vi "Read CAN Channels.vi"(7 "Peltier":T1, 8 "error in (no error)":errorcluster, 11 "Gas":T2) -> (0 "error out":errorcluster, 3 "CAN Values":dbl[](array[numeric]))   [LabVIEW 2014]
doc: "This VI is used as to not overload the CAN boards for acquiring data. The intent is to acquire one sample/second from the NI-DAQ hardware and one sample/5 seconds from the CAN boards. At the end of every 5 second cycle, fresh values are acquired. If in the middle of the 5 second wait, the last values are used. Please note that there is no timing inside this VI, it is solely dependent on the timing of the owning VI"
uses:
  CAN Communication/PAS/PAS.lvclass
  CAN Communication/PAS/Typedefs/Pressure Sensor.ctl
  CAN Communication/Peltier/Peltier.lvclass
  CAN Communication/Peltier/Typedefs/Peltier Temperature Sensors.ctl
  CAN Communication/PAS/Typedefs/Session Handle.ctl
  CAN Communication/Peltier/Typedefs/Session Handle.ctl
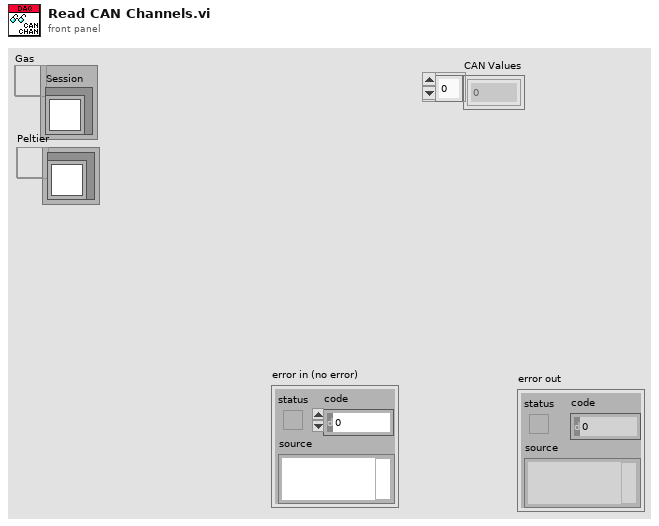
[diagram p1: front panel]
types:
  T1 = typedef "Peltier.lvclass/Session Handle.ctl" = refnum<data-value>
  T2 = typedef "PAS.lvclass/Session Handle.ctl" = refnum<data-value>
  T3 = typedef "Peltier.lvclass/Peltier Temperature Sensors.ctl" = u16
  T4 = typedef "PAS.lvclass/Pressure Sensor.ctl" = u16
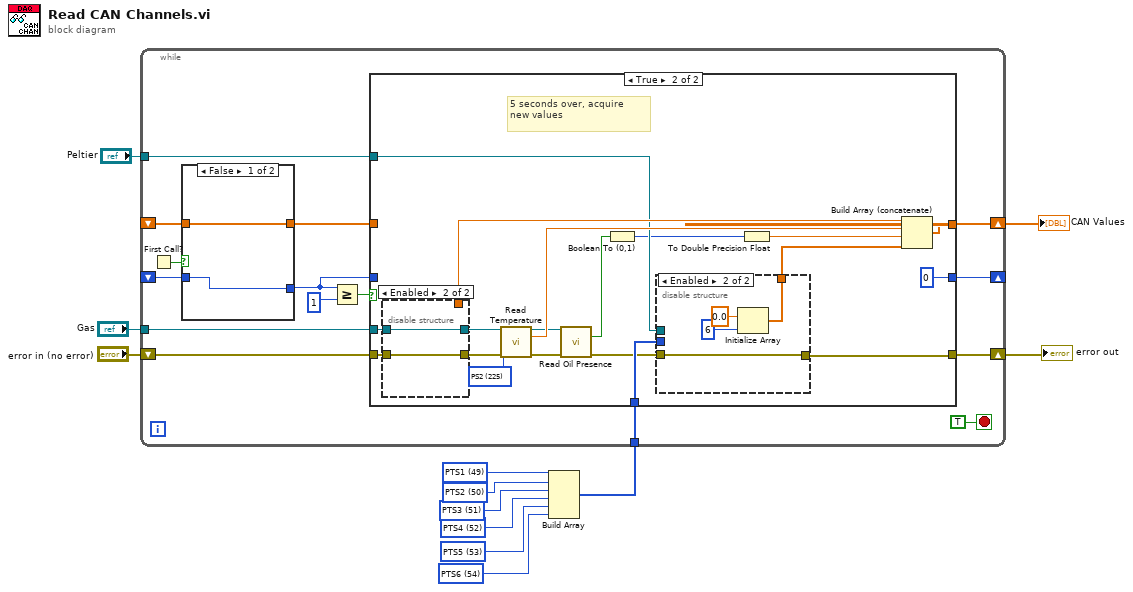
[diagram p0: block diagram]
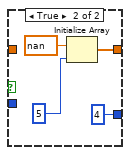
[diagram p2: hidden frame]
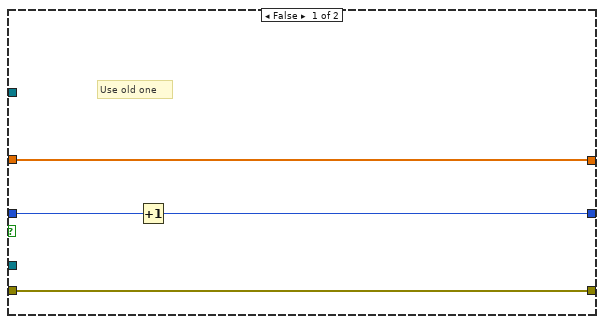
[diagram p3: hidden frame]
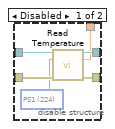
[diagram p4: hidden frame]
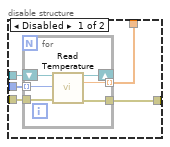
[diagram p5: hidden frame]
diagram:
  w2 = T3 54 items=["PTS1"=49, "PTS2"=50, "PTS3"=51, "PTS4"=52, "PTS5"=53, "PTS6"=54] ("Pelt Temp Sensors")
  w3 = T3 53 items=["PTS1"=49, "PTS2"=50, "PTS3"=51, "PTS4"=52, "PTS5"=53, "PTS6"=54] ("Pelt Temp Sensors")
  w4 = T3 52 items=["PTS1"=49, "PTS2"=50, "PTS3"=51, "PTS4"=52, "PTS5"=53, "PTS6"=54] ("Pelt Temp Sensors")
  w5 = T3 51 items=["PTS1"=49, "PTS2"=50, "PTS3"=51, "PTS4"=52, "PTS5"=53, "PTS6"=54] ("Pelt Temp Sensors")
  w6 = T3 50 items=["PTS1"=49, "PTS2"=50, "PTS3"=51, "PTS4"=52, "PTS5"=53, "PTS6"=54] ("Pelt Temp Sensors")
  w7 = T3 49 items=["PTS1"=49, "PTS2"=50, "PTS3"=51, "PTS4"=52, "PTS5"=53, "PTS6"=54] ("Pelt Temp Sensors")
  n1 = Build Array(w7, w6, w5, w4, w3, w2) -> (w1:T3[])
  n2 = while {
    tunnel: "Gas" -> [w23]
    shift-right: [w22] -> w10
    shift-left: _ -> [w19]
    shift-right: [w21] -> w9
    shift-left: "error in (no error)" -> [w24]
    shift-right: [w17] -> _
    shift-left: _ -> [w16]
    tunnel: "Peltier" -> [w14]
    tunnel: w1 -> [w13]
    stop <- TRUE stop-if-true
    n3 = First Call?() -> (First Call?: T/F=w20:bool)
    n4 = case shown="False" w20 {
      tunnel: [w29 w32] -> w15
      tunnel: [w28 4] -> w18
      tunnel: w19 -> [w29 _]
      tunnel: w16 -> [w28 _]
      frame False {
      }
      frame True {
        n5 = Initialize Array(nan ("element"), 5 ("dimension size")) -> (w32:dbl[])
      }
    }
    n6 = Greater Or Equal?(x=w18, y=1) -> (x >= y?=w26:bool)
    n7 = case shown="True" w26 {
      tunnel: w24 -> [w37 w56]
      tunnel: w23 -> [_ w55]
      tunnel: [w34 w49] -> w22
      tunnel: [w37 w45] -> w21
      tunnel: w18 -> [w36 _]
      tunnel: [w35 0] -> w17
      tunnel: w15 -> [w34 _]
      tunnel: w14 -> [_ w47]
      tunnel: w13 -> [_ w46]
      frame False {
        # "Use old one"
        n8 = Increment(x=w36) -> (x+1=w35:i32)
      }
      frame True {
        w52 = T4 225 items=["PS1"=224, "PS2"=225] ("Pressure Sensor")
        # "5 seconds over, acquire\nnew values"
        n9 = disable-structure shown="Enabled" {
          disable-tunnel: w56 -> [w62 w63]
          disable-tunnel: w55 -> [w60 w64]
          disable-tunnel: [w59 w63] -> w54
          disable-tunnel: [w58 w64] -> w53
          disable-tunnel: [w57 _] -> w51
          frame Disabled {
            w61 = T4 224 items=["PS1"=224, "PS2"=225] ("Pressure Sensor")
            n10 = call "Read Temperature.vi"("Session Handle in"=w60, 5:w61, "error in (no error)"=w62) -> ("Session Handle out"=w58:T2, "Temperature"=w57:dbl, "error out"=w59:errorcluster)  [unwired: 8 in, 2 out]
          }
          frame Enabled {
          }
        }
        n11 = call "Read Temperature.vi"("Session Handle in"=w53, 5:w52, "error in (no error)"=w54) -> ("Session Handle out"=w43:T2, "Temperature"=w50:dbl, "error out"=w44:errorcluster)  [unwired: 8 in, 2 out]
        n12 = call "Read Oil Presence.vi"("Session Handle in"=w43, "error in (no error)"=w44) -> ("Present?"=w40:bool, "error out"=w42:errorcluster)  [unwired: 11 in, 1 out]
        n13 = Boolean To (0,1)(Boolean=w40) -> (0, 1=w39:i16)
        n14 = disable-structure shown="Enabled" {
          disable-tunnel: w47 -> [w69 _]
          disable-tunnel: w46 -> [w68 _]
          disable-tunnel: [w67 w77] -> w45
          disable-tunnel: w42 -> [w66 w77]
          disable-tunnel: [w65 w76] -> w41
          frame Disabled {
            n15 = for {
              tunnel: w66 -> [w75]
              shift-right: [w73] -> _
              shift-left: w69 -> [w74]
              tunnel: [w72] -> w67
              tunnel: w68 -> [w71] mode=indexing
              tunnel: [w70] -> w65 mode=indexing
              n16 = call "Read Temperature.vi"("Session Handle"=w74, "Pelt Temp Sensors"=w71, "error in (no error)"=w75) -> ("Session Handle Out"=w73:T1, "Temperature"=w70:dbl, "error out"=w72:errorcluster)  [unwired: 10 in]
            }
          }
          frame Enabled {
            n17 = Initialize Array(0.0 ("element"), 6 ("dimension size")) -> (w76:dbl[])
          }
        }
        n18 = To Double Precision Float(number=w39) -> (double precision float=w38:dbl)
        n19 = Build Array (concatenate)(w51, w50, w38, w41) -> (w49:dbl[])
      }
    }
  }
  "error out" <- w9
  "CAN Values" <- w10
